vi "exceltolabview.vi"() -> ()   [LabVIEW 2018]
uses:
  <vilib>/Utility/NIReport.llb/Report Type.ctl
  <vilib>/addons/_office/excel.llb/Excel Get Data ([dbl]).vi
  <vilib>/Utility/NIReport.llb/NI_report.lvclass
  <vilib>/addons/_office/NI_ReportGenerationToolkit.lvlib
  <vilib>/Utility/NIReport.llb/NI_ReportGenerationCore.lvlib
  <vilib>/Utility/NIReport.llb/Excel/NI_Excel.lvclass
panel:
  out "输出数组 2":dbl[](array[numeric])
  out "data 2":dbl[][](array[numeric]) format="%.2f"
  in  "end (-1, -1) 2":cluster{"row":i32, "column":i32}={"row"=16, "column"=15}
  in  "start (-1, -1) 2":cluster{"row":i32, "column":i32}={"row"=16, "column"=0}
  out "输出数组":dbl[](array[numeric])
  out "data":dbl[][](array[numeric]) format="%.2f"
  out "4x4":T1
  in  "end (-1, -1)":cluster{"row":i32, "column":i32}={"row"=15, "column"=15}
  in  "start (-1, -1)":cluster{"row":i32, "column":i32}={"row"=15, "column"=0}
  out "初始化的数组":bool[](array[boolean])
  in  "template (empty)":path=path "C:/Users/86136/source/repos/data2.xlsx" caption="模板（空）"
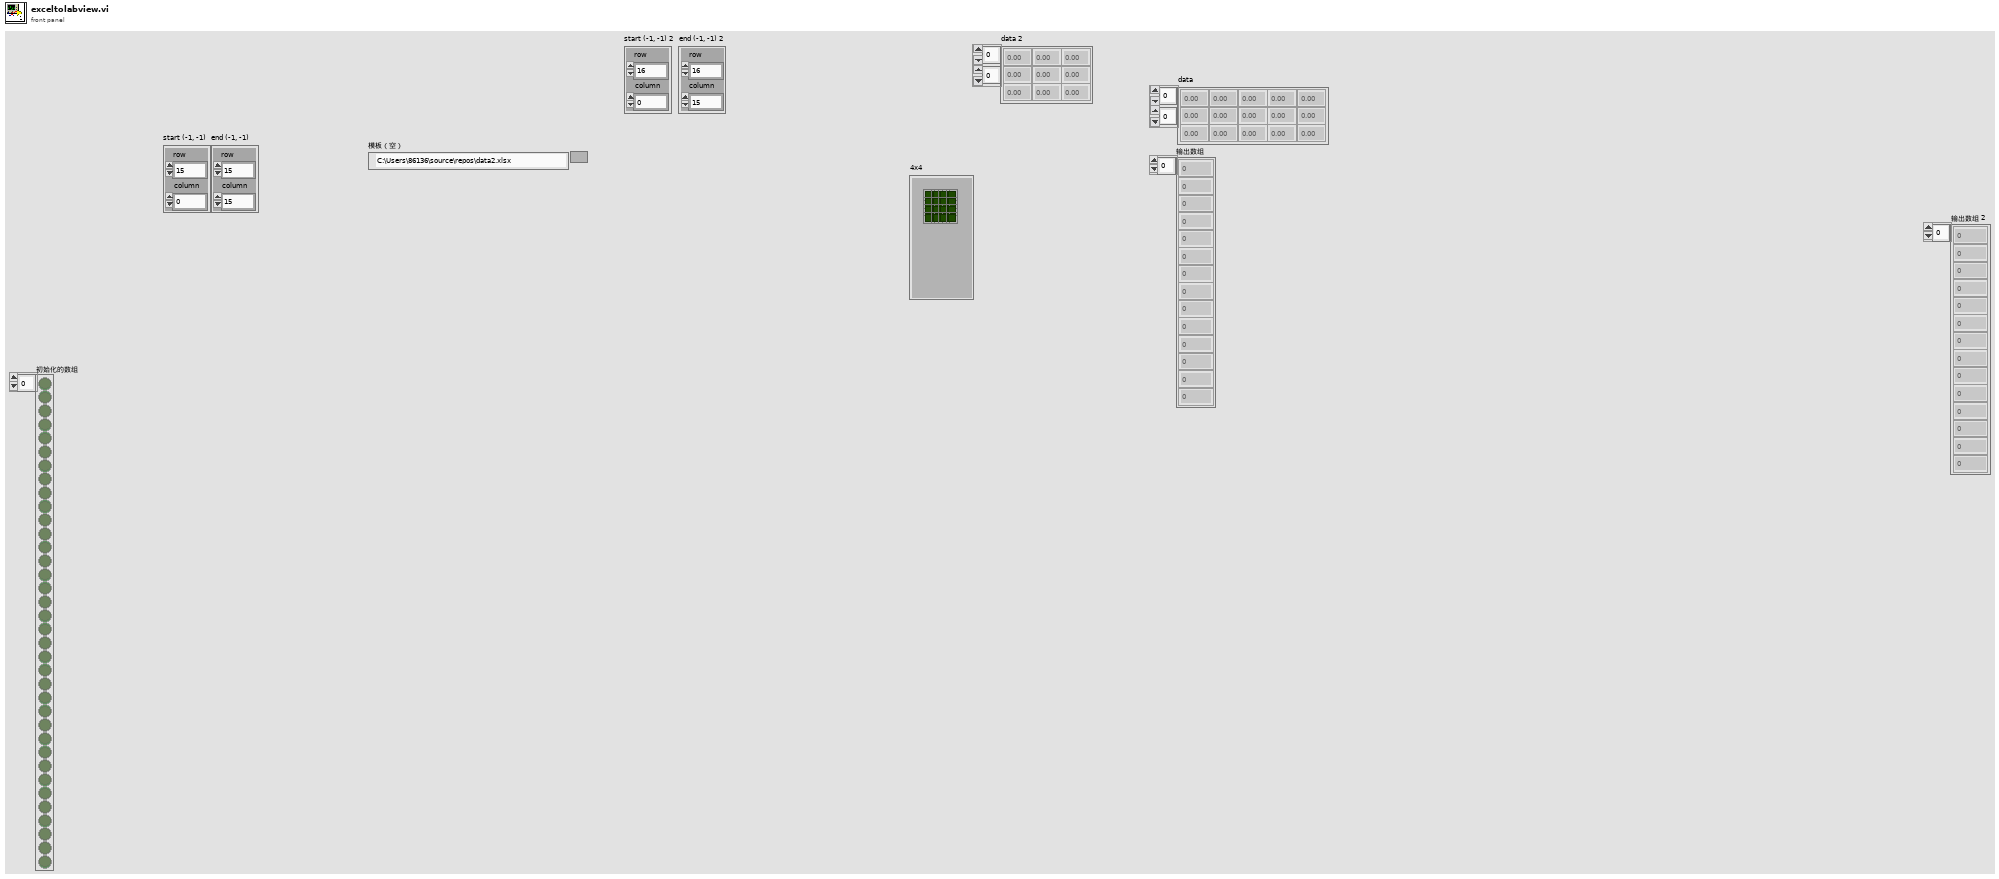
[diagram p1: front panel]
types:
  T1 = cluster{"布尔":bool, "布尔 2":bool, "布尔 3":bool, "布尔 4":bool, "布尔 5":bool, "布尔 6":bool, "布尔 7":bool, "布尔 8":bool, "布尔 9":bool, "布尔 10":bool, "布尔 11":bool, "布尔 12":bool, "布尔 13":bool, "布尔 14":bool, "布尔 15":bool, "布尔 16":bool}
  T2 = typedef "NI_ReportGenerationCore.lvlib/Report Type.ctl" = enum16{"HTML", "Word", "Excel"}
  T3 = enum16{"maximized", "minimized", "normal", "no change"}
  T4 = cluster{"[0]":bool, "[1]":bool, "[2]":bool, "[3]":bool, "[4]":bool, "[5]":bool, "[6]":bool, "[7]":bool, "[8]":bool, "[9]":bool, "[10]":bool, "[11]":bool, "[12]":bool, "[13]":bool, "[14]":bool, "[15]":bool}
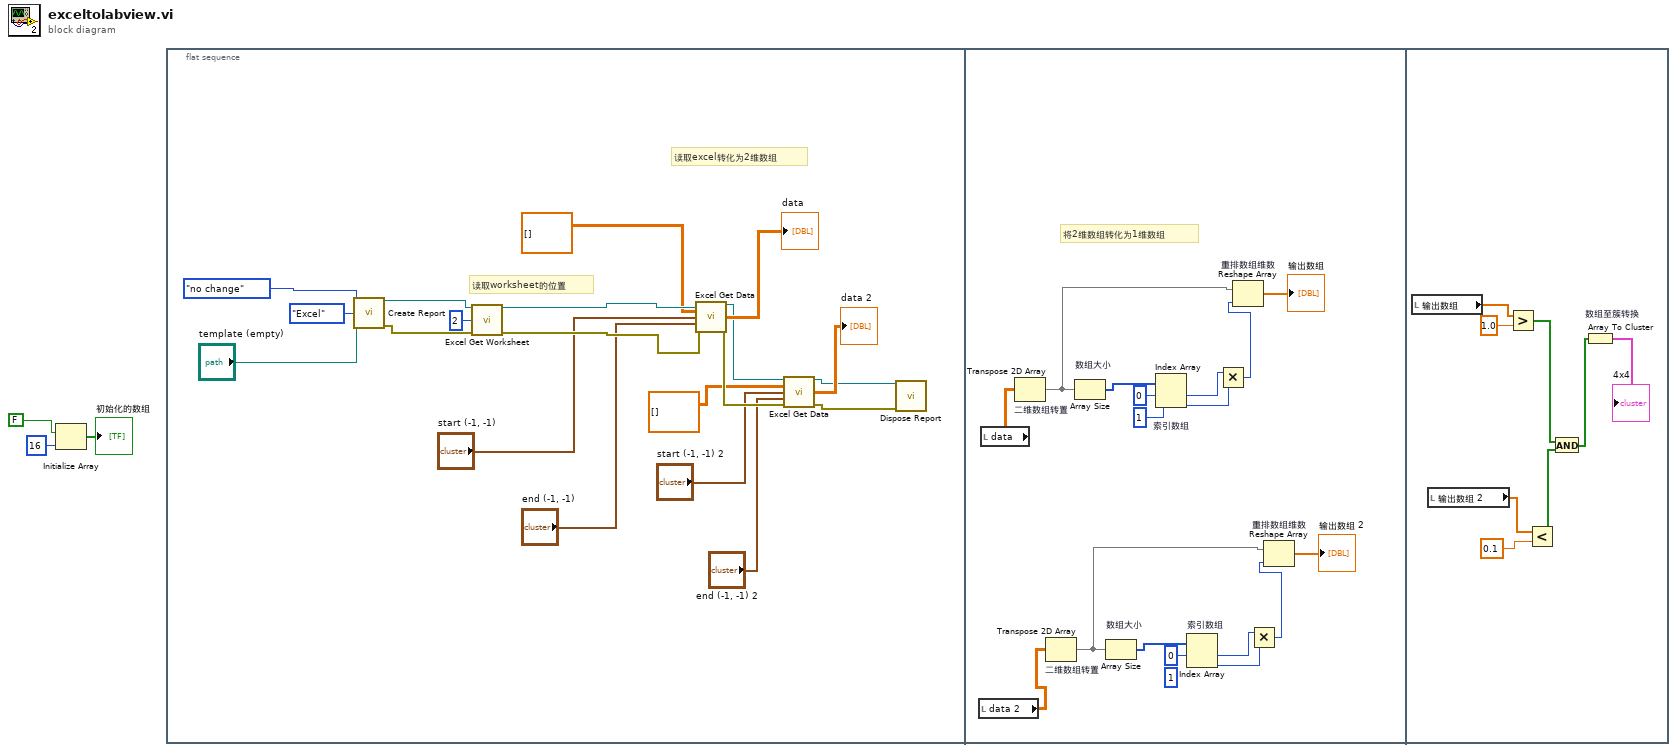
[diagram p0: block diagram]
diagram:
  n1 = Initialize Array(FALSE, 16 ("维数大小")) -> (→"初始化的数组":bool[])
  n2 = flat-sequence {
    frame #0 {
      # "读取worksheet的位置"
      # "读取excel转化为2维数组"
      n3 = call <vilib>:"Create Report.vi"("window state (normal)"=T3."no change", "report type"=Report_Type."Excel", "template (empty)"="template (empty)") -> ("report out"=w20:refnum<class "NI_report.lvclass">, "error out"=w19:errorcluster)  [unwired: 11 in]
      n4 = call <vilib>:"Excel Get Worksheet.vi"("report in"=w20, "worksheet index (0)"=2, "error in (no error)"=w19) -> ("report out"=w17:refnum<class "NI_report.lvclass">, "error out"=w16:errorcluster)  [unwired: 11 in]
      n5 = call-poly <vilib>:"Excel Get Data.vi"("report in"=w17, "data type"=dbl[][] [], "start (-1, -1)"="start (-1, -1)", "end (-1, -1)"="end (-1, -1)", "error in (no error)"=w16) -> ("report out"=w11:refnum<class "NI_report.lvclass">, "data"=→"data":dbl[][], "error out"=w10:errorcluster)  [unwired: 8 in]
      n6 = call-poly <vilib>:"Excel Get Data.vi"("report in"=w11, "data type"=dbl[][] [], "start (-1, -1)"="start (-1, -1) 2", "end (-1, -1)"="end (-1, -1) 2", "error in (no error)"=w10) -> ("report out"=w5:refnum<class "NI_report.lvclass">, "data"=→"data 2":dbl[][], "error out"=w4:errorcluster)  [unwired: 8 in]
      n7 = call-dynamic "Dispose Report.vi"("report in"=w5, "error in (no error)"=w4) -> ()  [unwired: 13 in, 1 out]
    }
    frame #1 {
      (unwired) 1 ("索引")
      # "将2维数组转化为1维数组"
      n8 = local read "data 2"() -> (w24:dbl[][])
      n9 = local read "data"() -> (w33:dbl[][])
      n10 = Transpose 2D Array "二维数组转置"(2D array=w33) -> (transposed array=w36:dbl[][])
      n11 = Transpose 2D Array "二维数组转置"(2D array=w24) -> (transposed array=w27:dbl[][])
      n12 = Array Size "数组大小"(array=w36) -> (size(s)=w37:i32[])
      n13 = Array Size "数组大小"(array=w27) -> (size(s)=w28:i32[])
      n14 = Index Array "索引数组"(array=w37, index #1=0 ("索引"), index #2=1 ("索引")) -> (element #1=w38:i32, element #2=w39:i32)
      n15 = Index Array "索引数组"(array=w28, index #1=0 ("索引")) -> (element #1=w29:i32, element #2=w30:i32)  [unwired: 1 in]
      n16 = Multiply(x=w38, y=w39) -> (x*y=w40:i32)
      n17 = Reshape Array "重排数组维数"(w36, w40) -> (→"输出数组":dbl[])
      n18 = Multiply(x=w29, y=w30) -> (x*y=w31:i32)
      n19 = Reshape Array "重排数组维数"(w27, w31) -> (→"输出数组 2":dbl[])
    }
    frame #2 {
      n20 = local read "输出数组"() -> (w47:dbl[])
      n21 = local read "输出数组 2"() -> (w44:dbl[])
      n22 = Greater?(x=w47, y=1.0) -> (0:w43:bool[])
      n23 = Less?(x=w44, y=0.1) -> (x < y?=w42:bool[])
      n24 = And(x=w43, y=w42) -> (x .and. y?=w41:bool[])
      n25 = Array To Cluster "数组至簇转换"(array=w41) -> (cluster=→"4x4":T4)
    }
  }
